vi "PPS_TRAJECTORY_EXECUTE_ABS.vi"(8 "Init":bool) -> (0 "AtReference":bool, 3 "Chassis Velocity Target SI":T1 {"vOmega" format="%10.3f"; "vY" format="%10.3f"; "vX" format="%10.3f"})   [LabVIEW 2019]
uses:
  <vilib>/Rock Robotics/WPI/ThirdParty/JAS_Junk/TrajLib/Trajectory_Library.lvlib
  CHS_TRAJECTORY_GLOBALS.vi
  <vilib>/Rock Robotics/WPI/ThirdParty/MJansen/PathPlanner/PathPlanner24.lvlib
  <vilib>/Rock Robotics/WPI/ThirdParty/ChoreoLib/ChoreoLib.lvlib
  <vilib>/Rock Robotics/WPI/ThirdParty/JAS_Junk/TrajLib/TypeDef/CHASSIS_SPEEDS.ctl
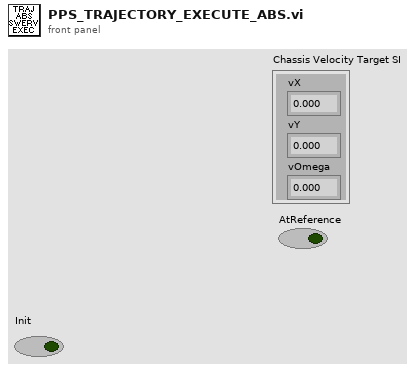
[diagram p1: front panel]
types:
  T1 = typedef "Trajectory_Library.lvlib/CHASSIS_SPEEDS.ctl" = cluster{"vX":dbl, "vY":dbl, "vOmega":dbl}
  T2 = typedef "Trajectory_Library.lvlib/POSE2D.ctl" = cluster{"TRANSLATION":T3, "ROTATION":T4}
  T3 = typedef "Trajectory_Library.lvlib/TRANSLATION2D.ctl" = cluster{"X":dbl, "Y":dbl}
  T4 = typedef "Trajectory_Library.lvlib/ROTATION2D.ctl" = cluster{"VALUE":dbl, "COS":dbl, "SIN":dbl}
  T5 = typedef "Trajectory_Library.lvlib/HOLONOMIC_DRV_CTRL.ctl" = cluster{"poseTolerance":T2, "poseError":T2, "Enabled":bool, "PID_xCtrl":T6, "PID_yCtrl":T6, "PROF_PID_thetaCtrl":T7, "RotationError":T4, "FirstRun":bool}
  T6 = typedef "Trajectory_Library.lvlib/PID_CONTROLLER.ctl" = cluster{"Kp":dbl, "Ki":dbl, "Kd":dbl, "Period":dbl, "Max_Integral":dbl, "Min_Integral":dbl, "Max_Input":dbl, "Min_Input":dbl, "Continuous":bool, "PositionError":dbl, "VelocityError":dbl, "PrevError":dbl, "TotalError":dbl, "PositionTolerance":dbl, "VelocityTolerance":dbl, "SetPoint":dbl, "Kf":dbl, "Prev_Deriv":dbl, "Prev_Deriv 2":dbl, "DerivativeFilter":bool, "Min_Output":dbl, "Max_Output":dbl, "Prev_F_P":dbl, "Prev_F_P_2":dbl, "AntiWindupActive":bool, "Measurement":dbl}
  T7 = typedef "Trajectory_Library.lvlib/PROFILED_PID_CONTROLLER.ctl" = cluster{"Controller":T6, "Goal":T8, "Setpoint":T8, "Constraint":T9}
  T8 = typedef "Trajectory_Library.lvlib/TRAPEZOID_PROFILE_STATE.ctl" = cluster{"Position":dbl, "Velocity":dbl}
  T9 = typedef "Trajectory_Library.lvlib/TRAPEZOID_PROFILE_CONSTRAINT.ctl" = cluster{"MaxVelocity":dbl, "MaxAcceleration":dbl}
  T10 = typedef "ChoreoLib.lvlib/ChoreoTrajectoryState.ctl" = cluster{"timestamp":dbl, "x":dbl, "y":dbl, "heading":dbl, "velocityX":dbl, "velocityY":dbl, "angularVelocity":dbl}
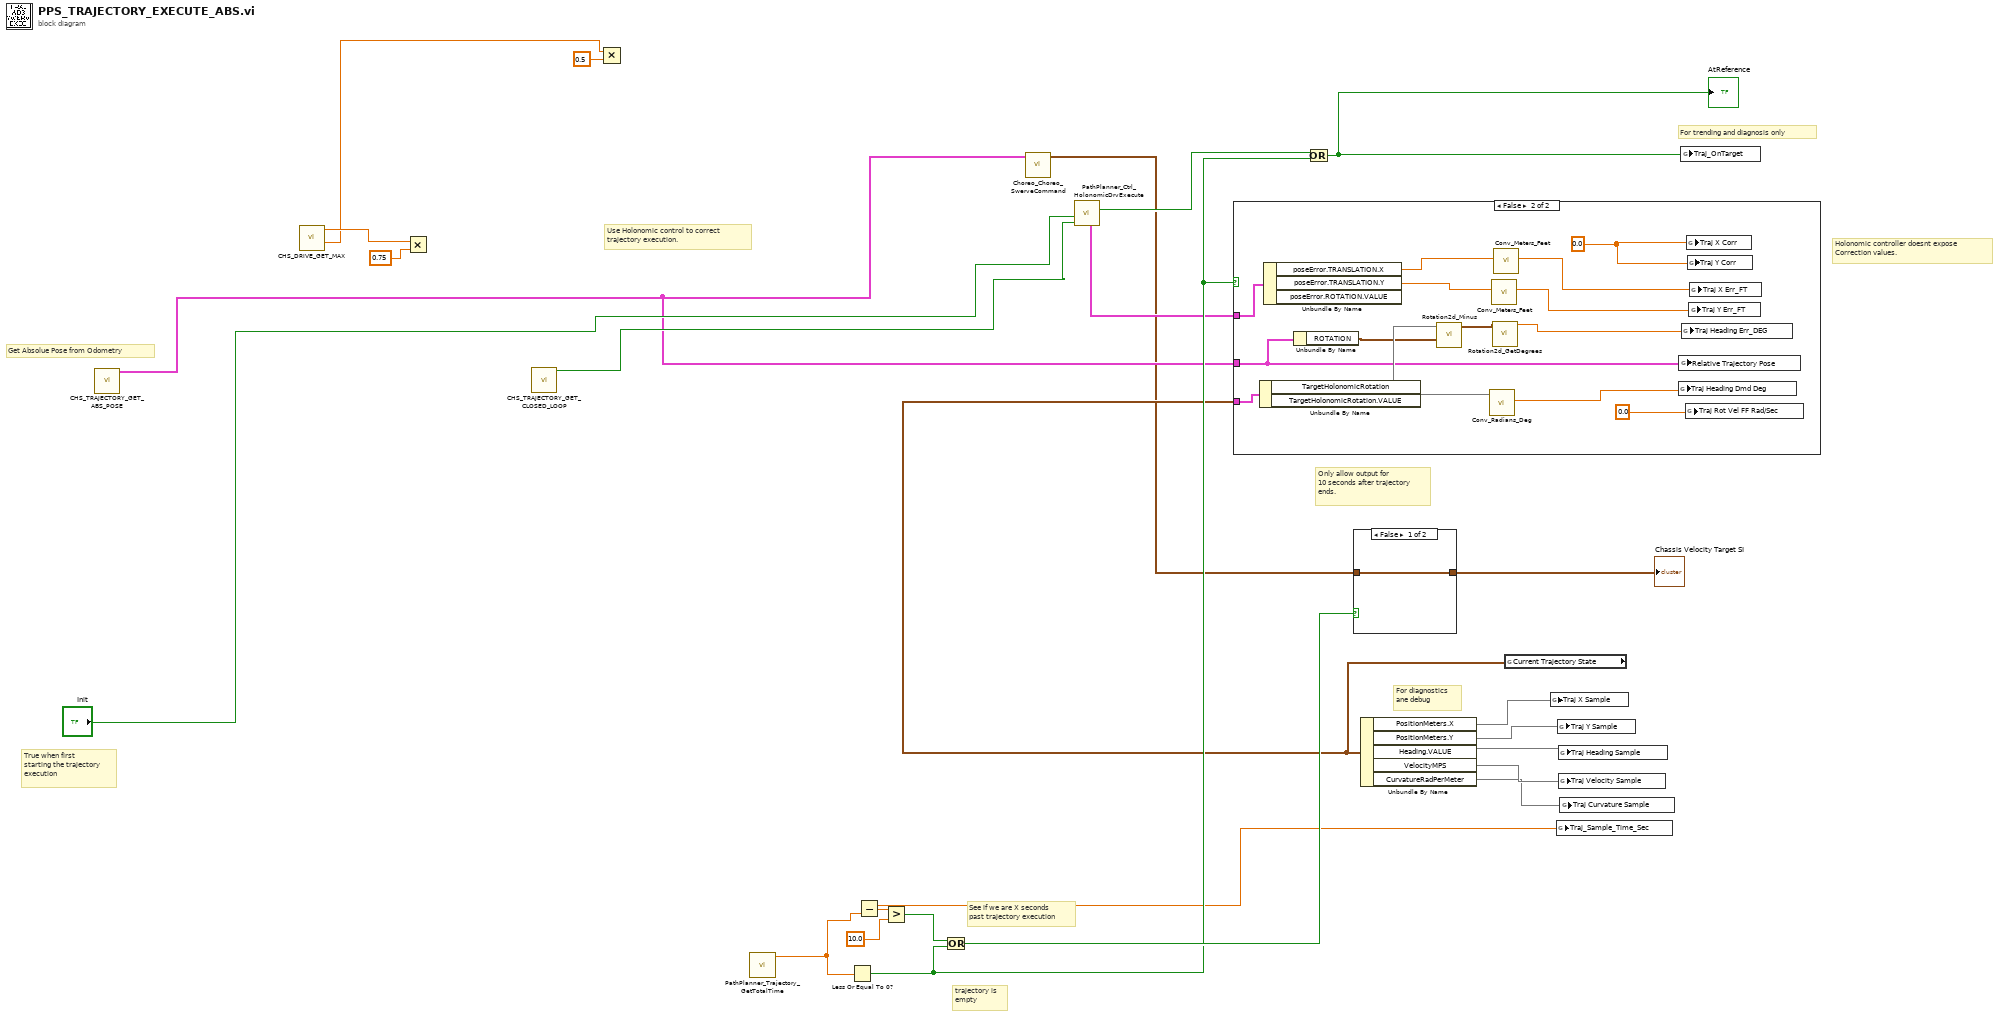
[diagram p0: block diagram]
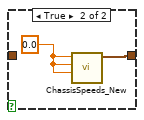
[diagram p3: hidden frame]
diagram:
  # "trajectory is \nempty"
  # "True when first\nstarting the trajectory\nexecution"
  # "Holonomic controller doesnt expose\nCorrection values."
  # "Use Holonomic control to correct\ntrajectory execution."
  # "For trending and diagnosis only"
  # "For diagnostics\nane debug"
  # "Get Absolue Pose from Odometry"
  # "See if we are X seconds \npast trajectory execution"
  # "Only allow output for\n10 seconds after trajectory\nends."
  n1 = call "CHS_TRAJECTORY_GET_ABS_POSE.vi"() -> ("Absolute Odometry Pose"=w2:T2)  [unwired: 11 in]
  n2 = call "CHS_DRIVE_GET_MAX.vi"() -> ("Max Rotational Vel (Rad/Sec)"=w6:dbl, "Max Wheel Vel (Meter/Sec)"=w8:dbl)  [unwired: 10 in]
  n3 = Multiply(x=w8, y=0.75) -> (x*y=w10:dbl)
  n4 = call "CHS_TRAJECTORY_GET_CLOSED_LOOP.vi"() -> ("AUTO_CLOSED_LOOP"=w3:bool)  [unwired: 11 in]
  n5 = Multiply(x=w6, y=0.5) -> ()  [unwired: 1 out]
  n6 = call <vilib>:"PathPlanner_Trajectory_GetTotalTime.vi"() -> ("TotalTimeSeconds"=w12:dbl)  [unwired: 11 in]
  n7 = Less Or Equal To 0?(x=w12) -> (x <= 0?=w15:bool)
  n8 = Subtract(y=w12) -> (x=w14:dbl, x-y=w26:dbl)
  n9 = Greater?(x=w26, y=10.0) -> (0:w18:bool)
  n10 = Or(x=w18, y=w15) -> (x .or. y?=w17:bool)
  n11 = call <vilib>:"Choreo_Choreo_SwerveCommand.vi"("Current Position"=w2) -> ("Chassis Speed Dmd"=w1:T1)  [unwired: 10 in]
  n12 = call <vilib>:"PathPlanner_Ctrl_HolonomicDrvExecute.vi"("Enabled"=w3, "Reset"="Init") -> ("At Reference"=w13:bool, "outHOLONOMIC_DRV_CTRL"=w7:T5)  [unwired: 6 in, 2 out]
  n13 = Or(x=w13, y=w15) -> (x .or. y?=w16:bool)
  "AtReference" <- w16
  n14 = case shown="False" w17 {
    tunnel: w1 -> [w27 _]
    tunnel: [w27 w28] -> w24
    frame False {
    }
    frame True {
      w29 = 0.0 ("vX")
      n15 = call <vilib>:"ChassisSpeeds_New.vi"("vAngular"=w29, "vY"=w29, "vX"=w29) -> ("CHASSIS"=w28:T1)  [unwired: 8 in]
    }
  }
  "Chassis Velocity Target SI" <- w24
  n16 = global read "CHS_TRAJECTORY_GLOBALS.vi" "Current Trajectory State"() -> (w11:T10)
  n17 = case shown="False" w15 {
    tunnel: w2 -> [_ w33]
    tunnel: w7 -> [_ w40]
    tunnel: w11 -> [_ w37]
    frame True {
    }
    frame False {
      w44 = 0.0 ("Y Corr")
      n18 = Unbundle By Name(w37) -> ("TargetHolonomicRotation"=w34, "TargetHolonomicRotation.VALUE"=w36)
      n19 = Unbundle By Name(w40) -> ("poseError.TRANSLATION.X"=w39:dbl, "poseError.TRANSLATION.Y"=w38:dbl)  [unwired: 1 out]
      n20 = Unbundle By Name(w33) -> ("ROTATION"=w32:T4)
      n21 = call <vilib>:"Rotation2d_Minus.vi"("other ROTATION"=w32, "in ROTATION"=w34) -> ("out ROTATION"=w31:T4)  [unwired: 9 in]
      n22 = call <vilib>:"Conv_Radians_Deg.vi"("Radians"=w36) -> ("Degrees"=w35:dbl)  [unwired: 10 in]
      n23 = call <vilib>:"Conv_Meters_Feet.vi"("Meters"=w38) -> ("Feet"=w43:dbl)  [unwired: 10 in]
      n24 = call <vilib>:"Rotation2d_GetDegrees.vi"("in ROTATION"=w31) -> ("AngleDegrees"=w30:dbl)  [unwired: 10 in]
      n25 = call <vilib>:"Conv_Meters_Feet.vi"("Meters"=w39) -> ("Feet"=w42:dbl)  [unwired: 10 in]
      n26 = global write "CHS_TRAJECTORY_GLOBALS.vi" "Traj Heading Dmd Deg"(w35) -> ()
      n27 = global write "CHS_TRAJECTORY_GLOBALS.vi" "Relative Trajectory Pose"(w33) -> ()
      n28 = global write "CHS_TRAJECTORY_GLOBALS.vi" "Traj Heading Err_DEG"(w30) -> ()
      n29 = global write "CHS_TRAJECTORY_GLOBALS.vi" "Traj Rot Vel FF Rad/Sec"(0.0 ("Traj Heading Dmd Deg")) -> ()
      n30 = global write "CHS_TRAJECTORY_GLOBALS.vi" "Traj X Corr"(w44) -> ()
      n31 = global write "CHS_TRAJECTORY_GLOBALS.vi" "Traj Y Corr"(w44) -> ()
      n32 = global write "CHS_TRAJECTORY_GLOBALS.vi" "Traj Y Err_FT"(w43) -> ()
      n33 = global write "CHS_TRAJECTORY_GLOBALS.vi" "Traj X Err_FT"(w42) -> ()
    }
  }
  n34 = Unbundle By Name(w11) -> ("PositionMeters.X"=w23, "PositionMeters.Y"=w22, "Heading.VALUE"=w21, "VelocityMPS"=w20, "CurvatureRadPerMeter"=w19)
  n35 = global write "CHS_TRAJECTORY_GLOBALS.vi" "Traj X Sample"(w23) -> ()
  n36 = global write "CHS_TRAJECTORY_GLOBALS.vi" "Traj_Sample_Time_Sec"(w14) -> ()
  n37 = global write "CHS_TRAJECTORY_GLOBALS.vi" "Traj Y Sample"(w22) -> ()
  n38 = global write "CHS_TRAJECTORY_GLOBALS.vi" "Traj Heading Sample"(w21) -> ()
  n39 = global write "CHS_TRAJECTORY_GLOBALS.vi" "Traj Velocity Sample"(w20) -> ()
  n40 = global write "CHS_TRAJECTORY_GLOBALS.vi" "Traj Curvature Sample"(w19) -> ()
  n41 = global write "CHS_TRAJECTORY_GLOBALS.vi" "Traj_OnTarget"(w16) -> ()
